vi "niScope Cal Adjust Offset Range.vi"(0 "instrument handle":refnum<k15>, 5 "channels":string, 7 "range (V)":dbl format="%.2f", 9 "stimulus":dbl format="%.2f", 11 "error in":errorcluster) -> (4 "instrument handle out":refnum<k15>, 15 "error out":errorcluster)   [LabVIEW 2011]
doc: "For the NI 5132/5133, this VI externally calibrates the vertical offset. Refer to the NI 5132/5133 Calibration Procedure for the appropriate stimulus voltages."
uses:
  niScope_32.dll
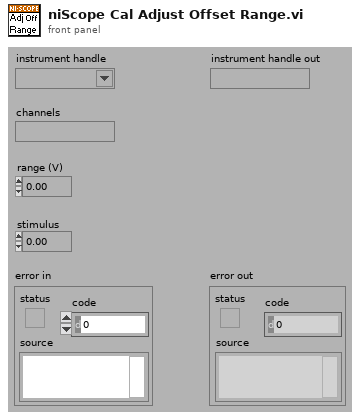
[diagram p1: front panel]
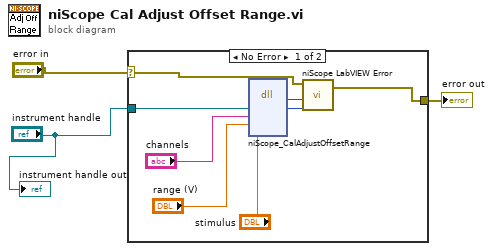
[diagram p0: block diagram]
diagram:
  n1 = case shown="No Error" "error in" {
    selector: "error in" -> [w4 w12]
    tunnel: [w5 w12] -> w3
    tunnel: "instrument handle" -> [w11 _]
    frame No Error {
      n2 = dll-call lib="niScope_*.*" fn="niScope_CalAdjustOffsetRange"("instrument handle"=w11, "Channel Name"="channels", "range"="range (V)", "stimulus"="stimulus") -> ("status"=w6:i32, "instrument handle"=w7:u32)  [unwired: 6 in, 2 out]
      n3 = call <instrlib>:"niScope LabVIEW Error.vi"("instrument handle"=w7, "niScope error code (0)"=w6, "error in (no error)"=w4) -> ("error out"=w5:errorcluster)  [unwired: 2 in]
    }
    frame Error {
    }
  }
  "error out" <- w3
  "instrument handle out" <- "instrument handle"
